vi "Export_2DtoTxt v10.6.0.vi"(0 "ITC503 Current Values":T4 {"ITC503 Gradient" format="%.2f"; "ITC503 Setpoint" min=-273.0 max=300000.0 step=0.0001 format="%.1f"; "ITC503 I" format="%_1f"; "ITC503 P" format="%_1f"; "ITC503 Temperature" min=0.0 max=1645.0 step=1e-05 format="%.2f"; "ITC503 Heater" min=0.0 max=100.0 step=0.01 scale=0.0..100.0}, 1 "iHR Current Values":T5={"iHR 550 Front Entrance"=0.0, "iHR550 Side Exit"=0.0, "iHR550 Wavelength"=897.9988, "iHR550 Exit Mirror"=2, "iHR550 Grating"="1", "Grating Index"=1} {"iHR550 Exit Mirror" items=["EntranceMirror", "ExitMirror", "Front", "Side"]}, 2 "CCD Temperature":dbl caption="Temp. (°C)" min=10.0 max=160.0 step=0.1 format="%.1f", 3 "CCD Area":T2={"XStart"=1, "YStart"=1, "XStop"=2048, "YStop"=512, "XBin"=1, "YBin"=1}, 4 "CCD ADC":u16(ring) caption="ADC Frequency" items=["20 kHz       ", " 1 MHz       ", " 1 MHz Ultra ", "500 kHz Wrap"], 5 "CCD Gain":u16(ring)=1 caption="Gain Mode" items=["High Light", "Best Dynamic Range", "High Sensitivity"], 6 "Auto?":bool, 7 "Drive Current Values":T6 {"Drive Z Position" min=-273.0 max=300000.0 step=0.0001 format="%.3f"; "Drive Y Position" min=-273.0 max=300000.0 step=0.0001 format="%.3f"; "Drive X Position" min=-273.0 max=300000.0 step=0.0001 format="%.3f"}, 8 "Export Type":string, 9 "Spectra Settings":T3={"Integration Time"=10.0, "Repetitions"=10, "Mapping Spectra"=TRUE} caption="Mapping Spectra Settings" {"Repetitions" min=1 max=100 step=1; "Integration Time" min=0.5 max=6000.0 step=1.0 format="%.1f"}, 10 "Filename":string, 11 "Data (2D)":dbl[][](array[numeric]), 12 "Auto Folder":path caption="Ausgewählter Pfad", 13 "Mapping Parameters":T1={"X Start Position"=0.0, "X Stop Position"=10.0, "Y Start Position"=0.0, "Y Stop Position"=10.0, "Step Size"=1.0} {"Step Size" min=0.1 max=30.0 step=0.1 format="%.1f"; "Y Stop Position" min=0.0 max=30.0 step=0.1 format="%.1f"; "Y Start Position" min=0.0 max=30.0 step=0.1 format="%.1f"; "X Stop Position" min=0.0 max=30.0 step=0.1 format="%.1f"; "X Start Position" min=0.0 max=30.0 step=0.1 format="%.1f"}) -> (14 "File Path":path)   [LabVIEW 2010]
uses:
  NPC3SG/TypeDefs/NPC3SG Current Values.ctl
  iHR550/TypeDefs/iHR Current Values.ctl
  ITC503/TypeDefs/ITC503 Current Values.ctl
  Mapping/TypeDefs/Mapping Spectra Params.ctl
  Symphony/TypeDefs/Symphony Area Format.ctl
  Mapping/TypeDefs/Mapping Drive Params.ctl
  <vilib>/Utility/file.llb/Write To Spreadsheet File (DBL).vi
panel:
  out "Headers":string
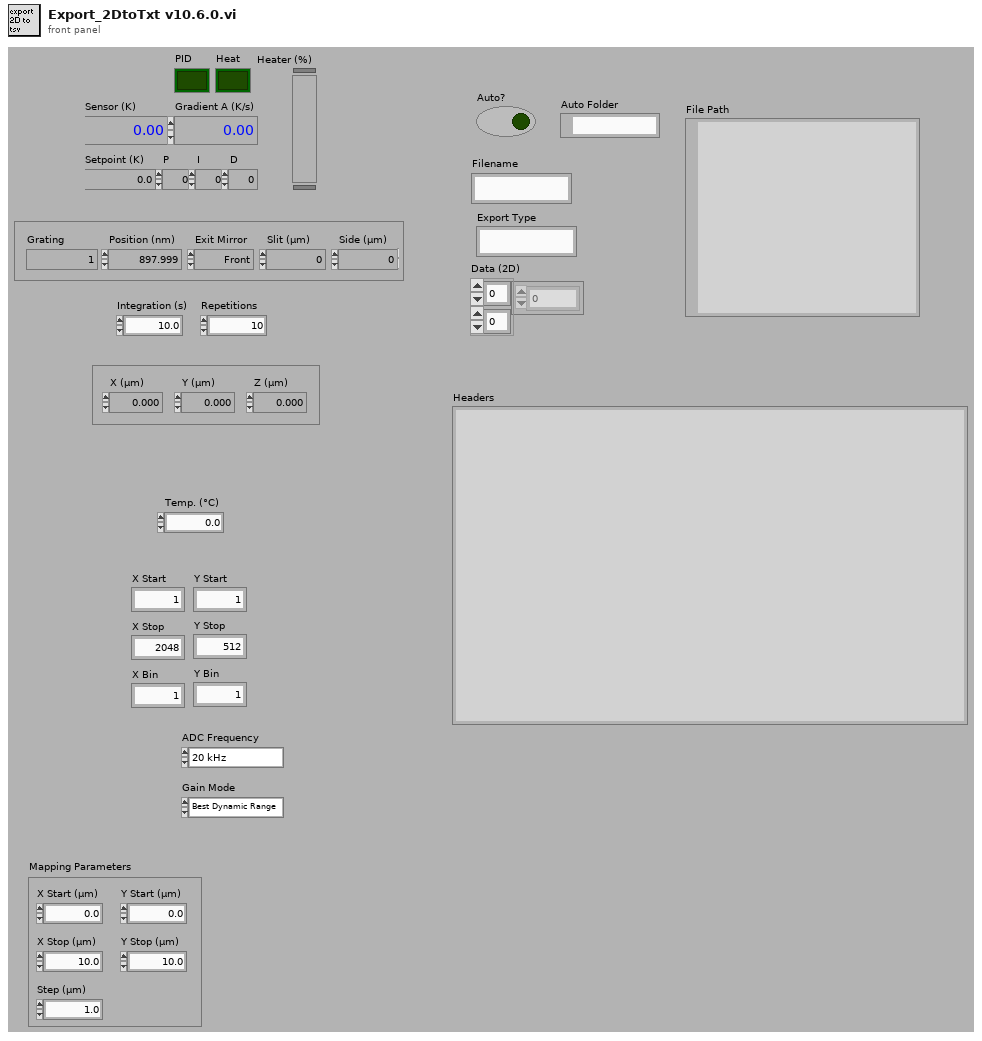
[diagram p1: front panel]
types:
  T1 = typedef "Mapping Drive Params.ctl" = cluster{"X Start Position":dbl, "X Stop Position":dbl, "Y Start Position":dbl, "Y Stop Position":dbl, "Step Size":dbl}
  T2 = typedef "Symphony Area Format.ctl" = cluster{"XStart":i32, "YStart":i32, "XStop":i32, "YStop":i32, "XBin":i32, "YBin":i32}
  T3 = typedef "Mapping Spectra Params.ctl" = cluster{"Integration Time":dbl, "Repetitions":u16, "Mapping Spectra":bool}
  T4 = typedef "ITC503 Current Values.ctl" = cluster{"ITC503 Heater":dbl, "ITC503 Temperature":dbl, "ITC503 P":dbl, "ITC503 I":dbl, "ITC503 D":dbl, "ITC503 Setpoint":dbl, "ITC503 Gradient":dbl, "ITC503 Heater Auto":bool, "ITC503 PID Auto":bool}
  T5 = typedef "iHR Current Values.ctl" = cluster{"iHR 550 Front Entrance":dbl, "iHR550 Side Exit":dbl, "iHR550 Wavelength":dbl, "iHR550 Exit Mirror":i32, "iHR550 Grating":string, "Grating Index":i32}
  T6 = typedef "NPC3SG Current Values.ctl" = cluster{"Drive X Position":dbl, "Drive Y Position":dbl, "Drive Z Position":dbl}
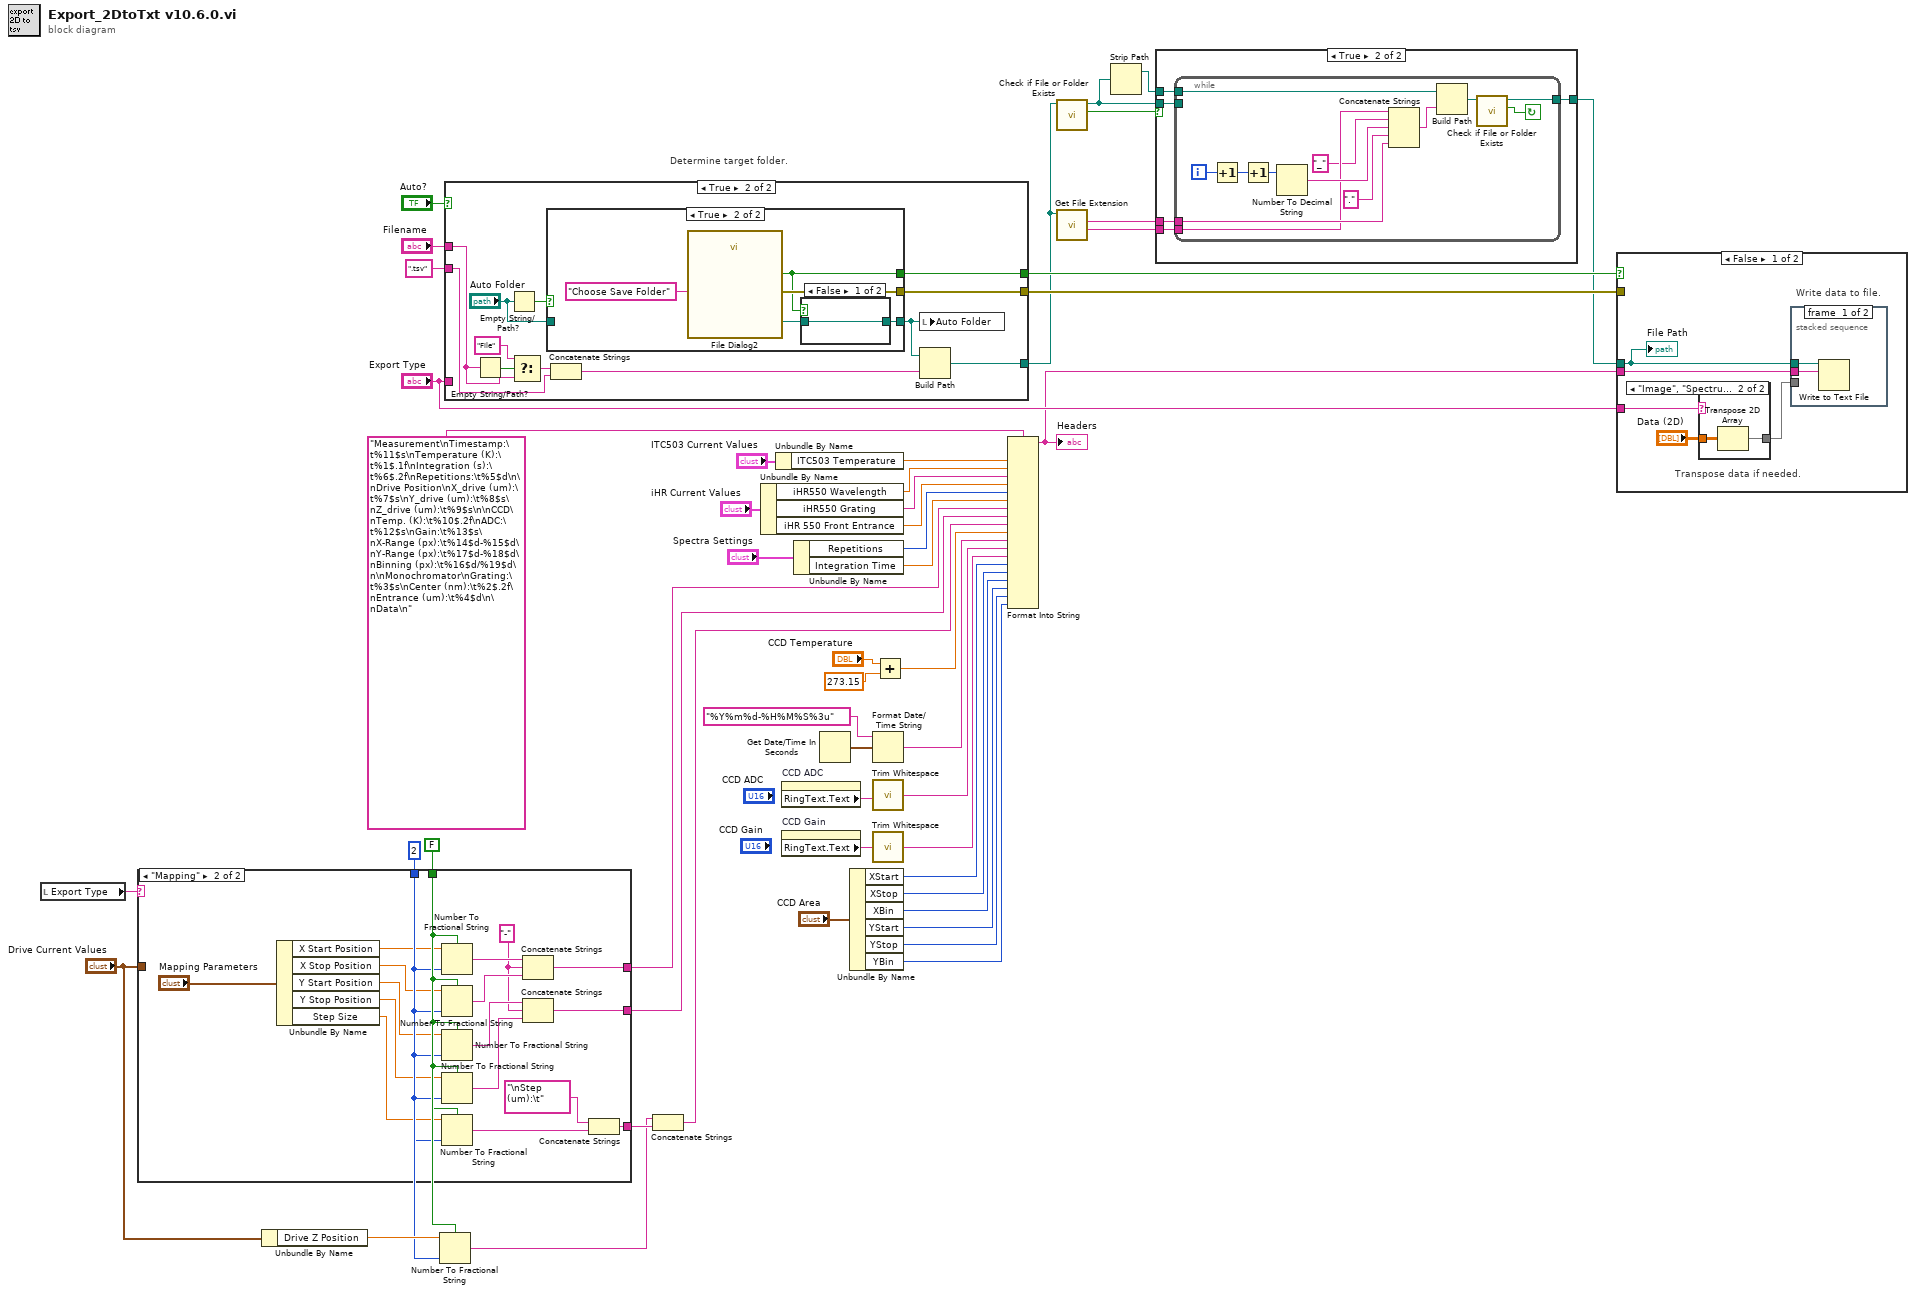
[diagram p0: block diagram]
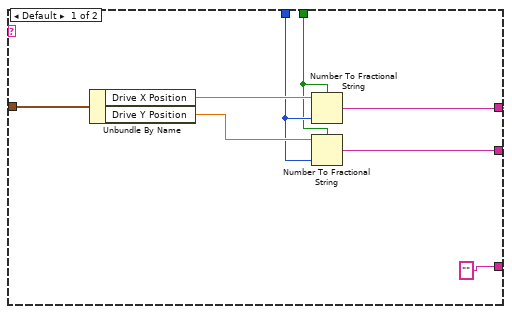
[diagram p2: hidden frame]
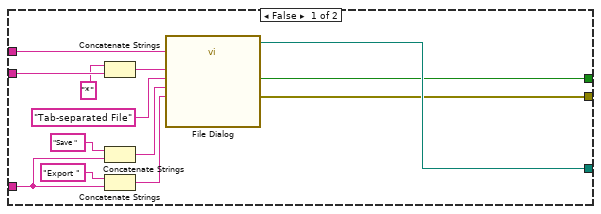
[diagram p4: hidden frame]
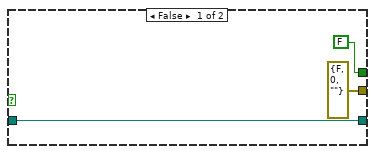
[diagram p5: hidden frame]
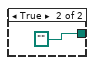
[diagram p6: hidden frame]
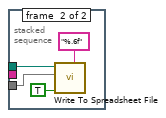
[diagram p7: hidden frame]
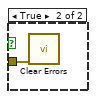
[diagram p9: hidden frame]
diagram:
  w5 = i16 2 ("precision (6)")
  w4 = FALSE ("use system decimal point (T)")
  # "Determine target folder."
  n1 = local read "Export Type"() -> (w10:string)
  n2 = case shown="\"Mapping\"" w10 {
    tunnel: [w57 w67] -> w9
    tunnel: [w56 w66] -> w8
    tunnel: "Drive Current Values" -> [w55 _]
    tunnel: w5 -> [w54 w65]
    tunnel: w4 -> [w53 w64]
    tunnel: ["" ("string") w60] -> w2
    frame Default {
      n3 = Unbundle By Name(w55) -> ("Drive X Position"=w59:dbl, "Drive Y Position"=w58:dbl)
      n4 = Number To Fractional String(use system decimal point (T)=w53, number=w59, precision (6)=w54) -> (F-format string=w57:string)  [unwired: 1 in]
      n5 = Number To Fractional String(use system decimal point (T)=w53, number=w58, precision (6)=w54) -> (F-format string=w56:string)  [unwired: 1 in]
    }
    frame "Mapping" {
      w68 = "-" ("string")
      n6 = Unbundle By Name("Mapping Parameters") -> ("X Start Position"=w76:dbl, "X Stop Position"=w75:dbl, "Y Start Position"=w74:dbl, "Y Stop Position"=w73:dbl, "Step Size"=w63:dbl)
      n7 = Number To Fractional String(use system decimal point (T)=w64, number=w76, precision (6)=w65) -> (F-format string=w72:string)  [unwired: 1 in]
      n8 = Number To Fractional String(use system decimal point (T)=w64, number=w75, precision (6)=w65) -> (F-format string=w71:string)  [unwired: 1 in]
      n9 = Number To Fractional String(use system decimal point (T)=w64, number=w74, precision (6)=w65) -> (F-format string=w70:string)  [unwired: 1 in]
      n10 = Number To Fractional String(use system decimal point (T)=w64, number=w73, precision (6)=w65) -> (F-format string=w69:string)  [unwired: 1 in]
      n11 = Number To Fractional String(use system decimal point (T)=w64, number=w63, precision (6)=w65) -> (F-format string=w61:string)  [unwired: 1 in]
      n12 = Concatenate Strings(w72, w68, w71) -> (w67:string)
      n13 = Concatenate Strings(w70, w68, w69) -> (w66:string)
      n14 = Concatenate Strings("\nStep (um):\t" ("string"), w61) -> (w60:string)
    }
  }
  n15 = Unbundle By Name("Drive Current Values") -> ("Drive Z Position"=w6:dbl)
  n16 = Number To Fractional String(use system decimal point (T)=w4, number=w6, precision (6)=w5) -> (F-format string=w1:string)  [unwired: 1 in]
  n17 = case shown="True" "Auto?" {
    tunnel: "Export Type" -> [w85 _]
    tunnel: [w84 w100] -> w14
    tunnel: [w83 w98] -> w49
    tunnel: [w82 w99] -> w48
    tunnel: ".tsv" ("pattern (all files)") -> [w80 w102]
    tunnel: "Filename" -> [w81 w96]
    frame False {
      n18 = Concatenate Strings("*" ("String"), w80) -> (w78:string)
      n19 = Concatenate Strings("Save " ("prompt"), w85) -> (w90:string)
      n20 = Concatenate Strings("Export " ("button label"), w85) -> (w89:string)
      n21 = call "File Dialog"("prompt"=w89, "button label"=w90, "default name"=w81, "pattern (all files)"=w78, "pattern label"="Tab-separated File") -> ("selected path"=w84:path, "cancelled"=w83:bool, "error out"=w82:errorcluster)  [unwired: 7 in, 1 out]
    }
    frame True {
      n22 = Empty String/Path?(string/path=w96) -> (empty?=w97:bool)
      n23 = Empty String/Path?(string/path="Auto Folder") -> (empty?=w92:bool)
      n24 = Select(t="File", s=w97, f=w96) -> (s? t:f=w94:string)
      n25 = case shown="True" w92 {
        tunnel: "Auto Folder" -> [w105 _]
        tunnel: [w105 w109] -> w91
        tunnel: [errorcluster {"status"=FALSE, "code"=0, "source"=""} ("error out") w108] -> w99
        tunnel: [FALSE ("cancelled") w107] -> w98
        frame False {
        }
        frame True {
          n26 = call "File Dialog2"("prompt"="Choose Save Folder") -> ("selected path"=w110:path, "cancelled"=w107:bool, "error out"=w108:errorcluster)  [unwired: 11 in, 1 out]
          n27 = case shown="False" w107 {
            tunnel: w110 -> [w111 _]
            tunnel: [w111 path ""] -> w109
            frame False {
            }
            frame True {
            }
          }
        }
      }
      n28 = Concatenate Strings(w94, w102) -> (w101:string)
      n29 = local write "Auto Folder"(w91) -> ()
      n30 = Build Path(base path=w91, name or relative path=w101) -> (appended path=w100:path)
    }
  }
  n31 = Concatenate Strings(w1, w2) -> (w3:string)
  n32 = Unbundle By Name("iHR Current Values") -> ("iHR550 Wavelength"=w40:dbl, "iHR550 Grating"=w39:string, "iHR 550 Front Entrance"=w38:dbl)
  n33 = Unbundle By Name("ITC503 Current Values") -> ("ITC503 Temperature"=w33:dbl)
  n34 = property on="CCD ADC" class="Ring (strict)"() -> ("RingText.Text"=w21:string)  [unwired: 2 in, 2 out]
  n35 = property on="CCD Gain" class="Ring (strict)"() -> ("RingText.Text"=w24:string)  [unwired: 2 in, 2 out]
  n36 = Unbundle By Name("Spectra Settings") -> ("Repetitions"=w37:u16, "Integration Time"=w36:dbl)
  n37 = Get Date/Time In Seconds() -> (seconds since 1Jan1904=w42:timestamp)
  n38 = Unbundle By Name("CCD Area") -> ("XStart"=w25:i32, "XStop"=w26:i32, "XBin"=w27:i32, "YStart"=w28:i32, "YStop"=w29:i32, "YBin"=w30:i32)
  n39 = Format Date/Time String(time format string (%c)="%Y%m%d-%H%M%S%3u", seconds (now)=w42) -> (date/time string=w35:string)  [unwired: 1 in]
  n40 = call <vilib>:"Trim Whitespace.vi"("string"=w21) -> ("trimmed string"=w22:string)  [unwired: 1 in]
  n41 = call <vilib>:"Trim Whitespace.vi"("string"=w24) -> ("trimmed string"=w23:string)  [unwired: 1 in]
  n42 = Add(x="CCD Temperature", y=273.15) -> (x+y=w18:dbl)
  n43 = Format Into String(format string="Measurement\nTimestamp:\t%11$s\nTemperature (K):\t%1$.1f\nIntegration (s):\t%6$.2f\nRepetitions:\t%5$d\n\nDrive Position\nX_drive (um):\t%7$s\nY_drive (um):\t%8$s\nZ_drive (um):\t%9$s\n\nCCD\nTemp. (K):\t%10$.2f\nADC:\t%12$s\nGain:\t%13$s\nX-Range (px):\t%14$d-%15$d\nY-Range (px):\t%17$d-%18$d\nBinning (px):\t%16$d/%19$d\n\nMonochromator\nGrating:\t%3$s\nCenter (nm):\t%2$.2f\nEntrance (um):\t%4$d\n\nData\n" ("String"), w33, w40, w39, w38, w37, w36, w9, w8, w3, w18, w35, w22, w23, w25, w26, w27, w28, w29, w30) -> (resulting string=w32:string)  [unwired: 2 in, 1 out]
  "Headers" <- w32
  n44 = call <vilib>:"Check if File or Folder Exists.vi"("path"=w14) -> ("file or folder exists?"=w17:bool, "dup path"=w12:path)  [unwired: 8 in, 1 out]
  n45 = call <vilib>:"Get File Extension.vi"("file"=w14) -> ("filename without extension"=w15:string, "lowercase file extension"=w16:string)  [unwired: 7 in, 2 out]
  n46 = Strip Path(path=w12) -> (stripped path=w11:path)  [unwired: 1 out]
  n47 = case shown="True" w17 {
    tunnel: [w113 w118] -> w13
    tunnel: w12 -> [w113 w117]
    tunnel: w16 -> [_ w116]
    tunnel: w15 -> [_ w115]
    tunnel: w11 -> [_ w114]
    frame False {
    }
    frame True {
      n48 = while {
        tunnel: w117 -> [_]
        tunnel: [w130] -> w118
        tunnel: w116 -> [w127]
        tunnel: w115 -> [w126]
        tunnel: w114 -> [w123]
        i -> [w120]
        stop <- w131 continue-if-true
        n49 = Increment(x=w120) -> (x+1=w119:i32)
        n50 = Increment(x=w119) -> (x+1=w128:i32)
        n51 = Number To Decimal String(number=w128) -> (decimal integer string=w129:string)  [unwired: 1 in]
        n52 = Concatenate Strings(w126, "_" ("string"), w129, "." ("string"), w127) -> (w122:string)
        n53 = Build Path(base path=w123, name or relative path=w122) -> (appended path=w121:path)
        n54 = call <vilib>:"Check if File or Folder Exists.vi"("path"=w121) -> ("file or folder exists?"=w131:bool, "dup path"=w130:path)  [unwired: 8 in, 1 out]
      }
    }
  }
  n55 = case shown="False" w49 {
    tunnel: w13 -> [w132 _]
    tunnel: w48 -> [_ w146]
    tunnel: "Export Type" -> [w135 _]
    tunnel: w32 -> [w134 _]
    frame False {
      # "Write data to file."
      # "Transpose data if needed."
      n56 = case shown="\"Image\", \"Spectrum\"" w135 {
        tunnel: "Data (2D)" -> [w143 w145]
        tunnel: [w143 w144] -> w133
        frame "Map", Default {
        }
        frame "Image", "Spectrum" {
          n57 = Transpose 2D Array(2D array=w145) -> (transposed array=w144:dbl[][])
        }
      }
      n58 = stacked-sequence {
        tunnel: w132 -> [w138 w139]
        tunnel: w134 -> [w137 _]
        tunnel: w133 -> [_ w140]
        frame #0 {
          n59 = Write to Text File(file (use dialog)=w138, text=w137) -> ()  [unwired: 2 in, 3 out]
        }
        frame #1 {
          n60 = call-poly <vilib>:"Write To Spreadsheet File.vi"("format (%.3f)"="%.6f", "append to file? (new file:F)"=TRUE, "2D data"=w140, "file path (dialog if empty)"=w139) -> ()  [unwired: 4 in, 1 out]
        }
      }
      "File Path" <- w132
    }
    frame True {
      n61 = call <vilib>:"Clear Errors.vi"("error in (no error)"=w146) -> ()  [unwired: 6 in, 1 out]
    }
  }
